vi "Regatron.G5.Rest VI Tree.vi"   [LabVIEW 2021, in "G5 Regatron Custom Device Shared.lvlib"]
doc: "The VI Tree displays all the user-callable VIs of the Regatron driver in an organized table."
uses:
  G5 Regatron Custom Device/Shared/G5 Regatron Custom Device Shared.lvlib
  Regatron.G5.Rest Protect Settings.llb/G5.Rest Protect Enable.vi
  Regatron.G5.Rest Datatypes.llb/G5.Rest Grid Values INT32.vi
panel:
  # "SEE DIAGRAM\nFOR VI TREE."
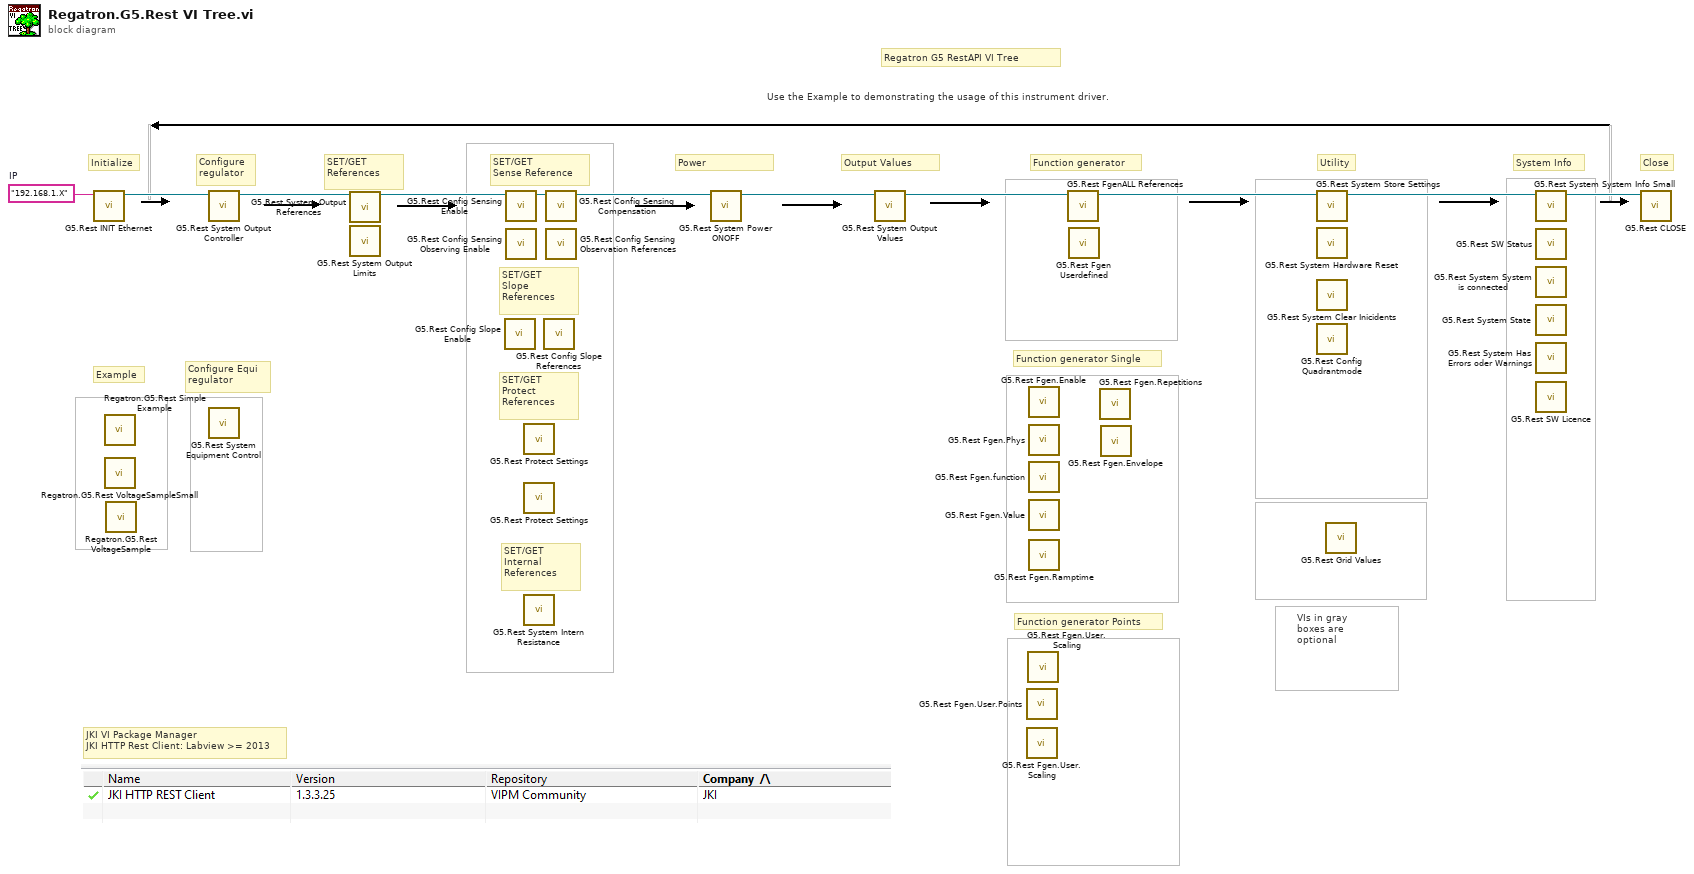
[diagram p0: block diagram]
diagram:
  w4 = "192.168.1.X"  # IP
  # "JKI VI Package Manager\nJKI HTTP Rest Client: Labview >= 2013"
  # "Function generator Points"
  # "Function generator Single"
  # "Function generator"
  # "Configure Equi\nregulator"
  # "SET/GET\nProtect\nReferences"
  # "SET/GET\nSlope\nReferences"
  # "SET/GET\nSense Reference"
  # "SET/GET\nInternal\nReferences"
  # "Power"
  # "System Info"
  # "Example"
  # "SET/GET\nReferences"
  # "Use the Example to demonstrating the usage of this instrument driver."
  # "VIs in gray\nboxes are\noptional"
  # "Regatron G5 RestAPI VI Tree"
  # "Configure\nregulator"
  # "Utility"
  # "Output Values"
  # "Close"
  # "Initialize"
  n1 = call "G5.Rest INIT Ethernet.vi"("IP"=w4) -> ("G5 WEB API"=w5:refnum<class "REST Client.lvclass">)  [unwired: 6 in, 4 out]
  n2 = call "Regatron.G5.Rest Simple Example.vi"() -> ()  [unwired: 12 in]
  n3 = call "Regatron.G5.Rest VoltageSampleSmall.vi"() -> ()  [unwired: 12 in]
  n4 = call "Regatron.G5.Rest VoltageSample.vi"() -> ()  [unwired: 12 in]
  n5 = call "G5.Rest System Output Controller.vi"("G5 WEB API (Eingang)"=w5) -> ("G5 WEB API (Ausgang)"=w11:refnum<class "REST Client.lvclass">)  [unwired: 8 in, 2 out]
  n6 = call "G5.Rest System Equipment Control.vi"() -> ()  [unwired: 9 in, 3 out]
  n7 = call "G5.Rest System Output References .vi"("G5 WEB API (Eingang)"=w11) -> ("G5 WEB API (Ausgang)"=w8:refnum<class "REST Client.lvclass">)  [unwired: 12 in, 2 out]
  n8 = call "G5.Rest System Output Limits.vi"() -> ()  [unwired: 13 in, 3 out]
  n9 = call "G5.Rest Config Slope Enable.vi"() -> ()  [unwired: 13 in, 3 out]
  n10 = call "G5.Rest Config Sensing Enable.vi"("G5 WEB API (Eingang)"=w8) -> ("G5 WEB API (Ausgang)"=w3:refnum<class "REST Client.lvclass">)  [unwired: 8 in, 2 out]
  n11 = call "G5.Rest Config Sensing Observing Enable.vi"() -> ()  [unwired: 9 in, 3 out]
  n12 = call-poly "G5.Rest Protect Settings.vi"() -> ()  [unwired: 13 in, 3 out]
  n13 = call-poly "G5.Rest Protect Settings.vi"() -> ()  [unwired: 13 in, 3 out]
  n14 = call "G5.Rest System Intern Resistance.vi"() -> ()  [unwired: 9 in, 3 out]
  n15 = call "G5.Rest Config Slope References.vi"() -> ()  [unwired: 13 in, 3 out]
  n16 = call "G5.Rest Config Sensing Compensation.vi"("G5 WEB API (Eingang)"=w3) -> ("G5 WEB API (Ausgang)"=w7:refnum<class "REST Client.lvclass">)  [unwired: 8 in, 2 out]
  n17 = call "G5.Rest Config Sensing Observation References.vi"() -> ()  [unwired: 13 in, 3 out]
  n18 = call "G5.Rest System Power ONOFF.vi"("G5 WEB API (Eingang)"=w7) -> ("G5 WEB API (Ausgang)"=w10:refnum<class "REST Client.lvclass">)  [unwired: 8 in, 2 out]
  n19 = call "G5.Rest System Output Values.vi"("G5 WEB API (Eingang)"=w10) -> ("G5 WEB API (Ausgang)"=w1:refnum<class "REST Client.lvclass">)  [unwired: 8 in, 2 out]
  n20 = call "G5.Rest Fgen.User.Points.vi"() -> ()  [unwired: 9 in, 3 out]
  n21 = call "G5.Rest Fgen.User.Scaling.vi"() -> ()  [unwired: 9 in, 3 out]
  n22 = call "G5.Rest Fgen.User.Scaling.vi"() -> ()  [unwired: 9 in, 3 out]
  n23 = call "G5.Rest Fgen.Enable.vi"() -> ()  [unwired: 9 in, 3 out]
  n24 = call "G5.Rest Fgen.Phys.vi"() -> ()  [unwired: 9 in, 3 out]
  n25 = call "G5.Rest Fgen.function.vi"() -> ()  [unwired: 9 in, 3 out]
  n26 = call "G5.Rest Fgen.Value.vi"() -> ()  [unwired: 9 in, 3 out]
  n27 = call "G5.Rest Fgen.Ramptime.vi"() -> ()  [unwired: 9 in, 3 out]
  n28 = call "G5.Rest FgenALL References .vi"("G5 WEB API (Eingang)"=w1) -> ("G5 WEB API (Ausgang)"=w6:refnum<class "REST Client.lvclass">)  [unwired: 8 in, 2 out]
  n29 = call "G5.Rest Fgen Userdefined .vi"() -> ()  [unwired: 9 in, 3 out]
  n30 = call "G5.Rest Fgen.Repetitions.vi"() -> ()  [unwired: 9 in, 3 out]
  n31 = call "G5.Rest Fgen.Envelope.vi"() -> ()  [unwired: 9 in, 3 out]
  n32 = call "G5.Rest System Store Settings.vi"("G5 WEB API (Eingang)"=w6) -> ("G5 WEB API (Ausgang)"=w2:refnum<class "REST Client.lvclass">)  [unwired: 9 in, 1 out]
  n33 = call "G5.Rest System Hardware Reset.vi"() -> ()  [unwired: 10 in, 2 out]
  n34 = call "G5.Rest System Clear Inicidents.vi"() -> ()  [unwired: 10 in, 2 out]
  n35 = call "G5.Rest Config Quadrantmode.vi"() -> ()  [unwired: 9 in, 3 out]
  n36 = call-poly "G5.Rest Grid Values.vi"() -> ()  [unwired: 9 in, 3 out]
  n37 = call "G5.Rest System System Info Small.vi"("G5 WEB API (Eingang)"=w2) -> ("G5 WEB API (Ausgang)"=w9:refnum<class "REST Client.lvclass">)  [unwired: 8 in, 2 out]
  n38 = call "G5.Rest SW Status.vi"() -> ()  [unwired: 9 in, 3 out]
  n39 = call "G5.Rest System System is connected.vi"() -> ()  [unwired: 9 in, 3 out]
  n40 = call "G5.Rest System State.vi"() -> ()  [unwired: 9 in, 3 out]
  n41 = call "G5.Rest System Has Errors oder Warnings.vi"() -> ()  [unwired: 7 in, 5 out]
  n42 = call "G5.Rest SW Licence.vi"() -> ()  [unwired: 9 in, 3 out]
  n43 = call "G5.Rest CLOSE.vi"("G5 WEB API"=w9) -> ()  [unwired: 10 in, 1 out]
